vi "GetChanName.vi"(8 "error in":errorcluster, 10 "Channel number":i32=1 min=1 max=28 step=1, 11 "VISA resource name":refnum<visa-resource-name>) -> (0 "error out":errorcluster, 2 "Name of channel":string, 3 "VISA resource name out":refnum<visa-resource-name>)   [LabVIEW 2023, in "Thermotron 8800.lvlib"]
doc: "CNAM\nCommand name: Get name of channel\nCommand type: System status\nDescription: This command allows you read the assigned name of any process variable or monitor\nchannel.\nSyntax: CNAMn?\nWhere n = channel number (1-12 are process variable channels, 13-28 are monitor\nchannels)\nData type: ASCII units character\nQuery example: CNAM10?\n8800 response: PROD MON"
uses:
  Thermotron 8800.lvlib
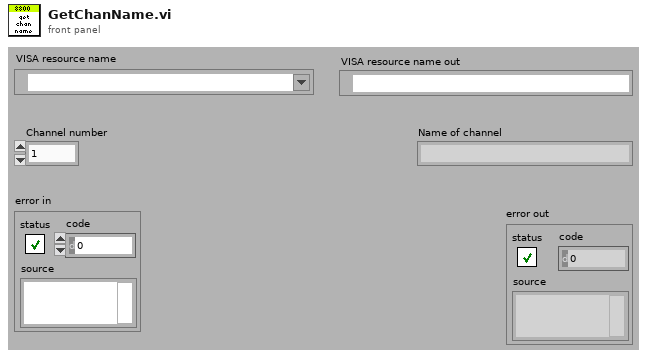
[diagram p1: front panel]
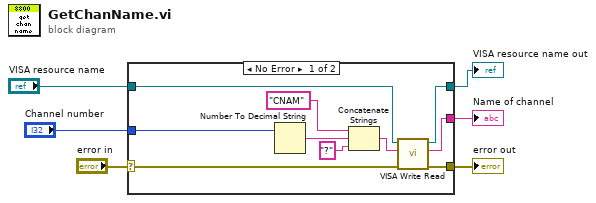
[diagram p0: block diagram]
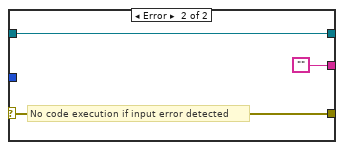
[diagram p2: hidden frame]
diagram:
  n1 = case shown="No Error" "error in" {
    selector: "error in" -> [w12 w19]
    tunnel: [w11 w19] -> w5
    tunnel: "Channel number" -> [w10 _]
    tunnel: "VISA resource name" -> [w9 w18]
    tunnel: [w8 w18] -> w2
    tunnel: [w7 ""] -> w1
    frame No Error {
      n2 = Number To Decimal String(number=w10) -> (decimal integer string=w15:string)  [unwired: 1 in]
      n3 = Concatenate Strings("CNAM" ("string"), w15, "?" ("string")) -> (w13:string)
      n4 = call "VISA Write Read.vi"("error in (no error)"=w12, "8800 Command"=w13, "VISA Refnum in"=w9) -> ("error out"=w11:errorcluster, "read buffer"=w7:string, "VISA Refnum out"=w8:refnum<visa-resource-name>)  [unwired: 6 in]
    }
    frame Error {
      # "No code execution if input error detected"
    }
  }
  "error out" <- w5
  "VISA resource name out" <- w2
  "Name of channel" <- w1
